vi "Cell color by inspection (2D).vi"(8 "에러 입력(에러 없음)":errorcluster, 9 "테이블 입력":refnum<vi>, 11 "Spec":string[][](array[string])) -> (0 "에러 출력":errorcluster, 1 "Data(DBL)":dbl[][](array[numeric]), 3 "Data(str)":string[][](array[string]))   [LabVIEW 2020]
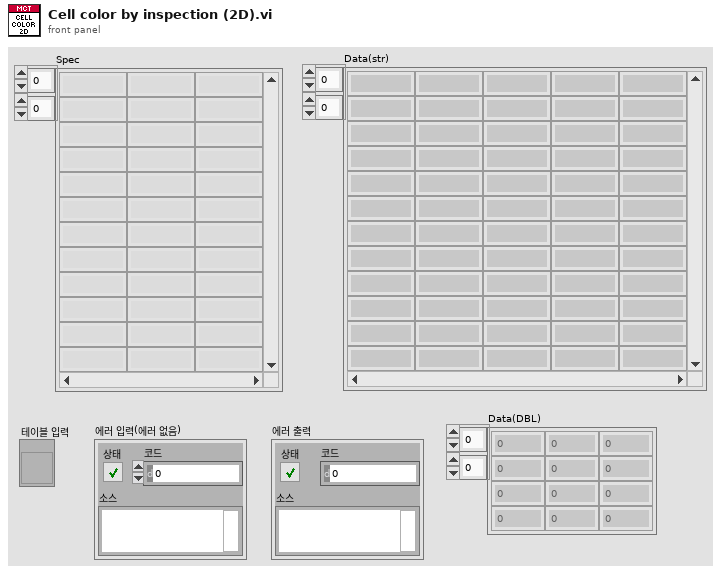
[diagram p1: front panel]
types:
  T1 = enum8{"Enabled", "Disabled", "Disabled and Grayed Out"}
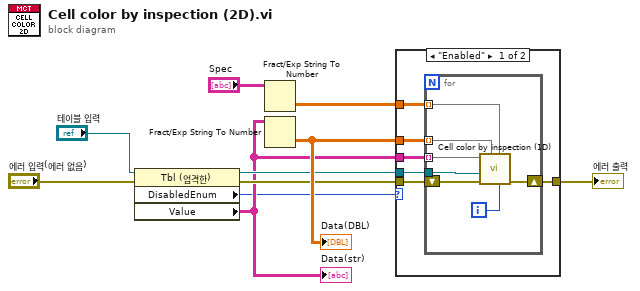
[diagram p0: block diagram]
diagram:
  n1 = property class="Tbl (엄격한)"(reference="테이블 입력", error in="에러 입력(에러 없음)") -> (reference out=w3:refnum<vi>, error out=w5:errorcluster, "DisabledEnum"=w1:T1, "Value"=w2:string[][])
  "Data(str)" <- w2
  n2 = Fract/Exp String To Number(string="Spec") -> (number=w7:dbl[][])  [unwired: 3 in, 1 out]
  n3 = Fract/Exp String To Number(string=w2) -> (number=w8:dbl[][])  [unwired: 3 in, 1 out]
  "Data(DBL)" <- w8
  n4 = case shown="\"Enabled\"" w1 {
    tunnel: [w16 w24] -> w10
    tunnel: w8 -> [w15 _]
    tunnel: w7 -> [w14 _]
    tunnel: w5 -> [w13 w24]
    tunnel: w3 -> [w12 _]
    tunnel: w2 -> [w11 _]
    frame "Enabled" {
      n5 = for {
        tunnel: w14 -> [w18] mode=indexing
        tunnel: w15 -> [w19] mode=indexing
        tunnel: w12 -> [w20]
        tunnel: w11 -> [w21] mode=indexing
        shift-right: [w22] -> w16
        shift-left: w13 -> [w23]
        i -> [w17]
        n6 = call "Cell color by inspection (1D).vi"("행번호"=w17, "Spec"=w18, "Data (DBL)"=w19, "에러 입력"=w23, "테이블 입력"=w20, "Data (str)"=w21) -> ("에러 출력"=w22:errorcluster)  [unwired: 5 in]
      }
    }
    frame Default {
    }
  }
  "에러 출력" <- w10
